vi "Write Faults Tab.vi"(8 "error in (no error)":errorcluster, 10 "Faults Tab":refnum<vi>, 11 "Fault Handler in":refnum<class "Fault Handler.lvclass">) -> (0 "error out":errorcluster, 3 "Fault Handler out":refnum<class "Fault Handler.lvclass">)   [LabVIEW 2023, in "Fault Handler.lvlib" / "Fault Handler.lvclass"]
uses:
  Library/Fault Handler.lvclass
  Library/Fault Handler.lvclass/Fault Handler.ctl
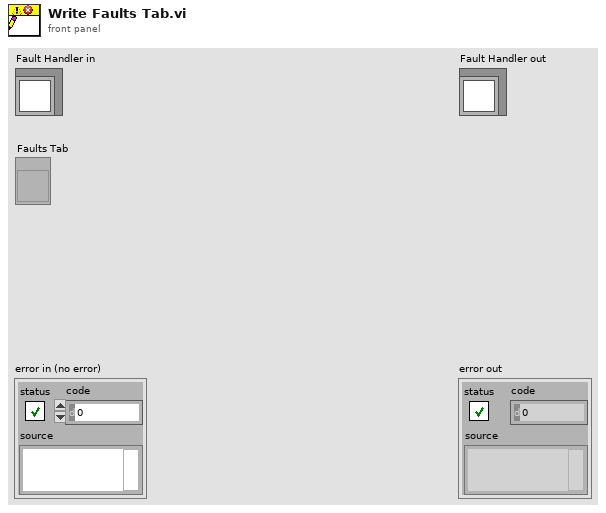
[diagram p1: front panel]
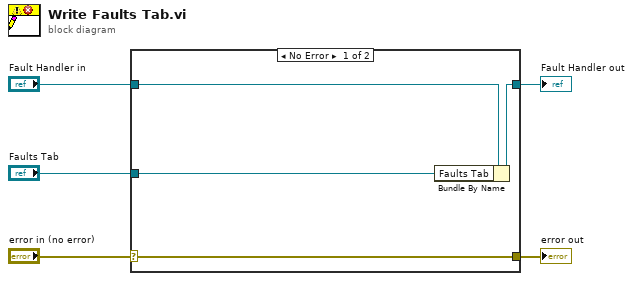
[diagram p0: block diagram]
diagram:
  n1 = case shown="No Error" "error in (no error)" {
    selector: "error in (no error)" -> [w9 w10]
    tunnel: [w9 w10] -> w4
    tunnel: [w7 w11] -> w2
    tunnel: "Fault Handler in" -> [w8 w11]
    tunnel: "Faults Tab" -> [w6 _]
    frame No Error {
      n2 = Bundle By Name(cluster=w8, "Faults Tab"=w6) -> (w7:refnum<class "Fault Handler.lvclass">)
    }
    frame Error {
    }
  }
  "error out" <- w4
  "Fault Handler out" <- w2
